vi "receiveTelemetry.vi"(8 "error in (no error)":errorcluster, 10 "tel connection in":refnum<k5>, 11 "TcpServer out":refnum<class "TcpServer.lvclass">) -> (0 "error out":errorcluster, 1 "telemetry received":string[](array[string]), 2 "tel connection out":refnum<k5>, 3 "tcpServer out":refnum<class "TcpServer.lvclass">)   [LabVIEW 2018]
doc: "Generate 50 elements and send them as telemetry to TCP client, and then read it."
uses:
  src/TcpServer/TcpServer.lvclass
  src/TcpServerTel/typedef/telTypeDef.ctl
  src/TcpServerTel/TcpServerTel.lvclass
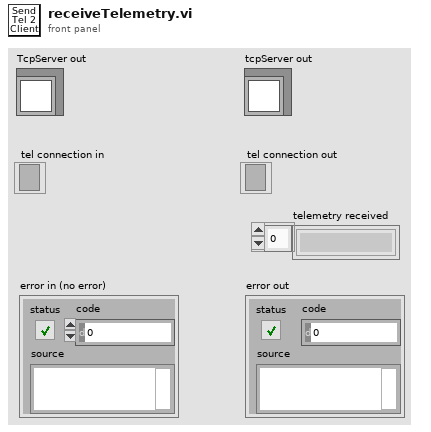
[diagram p1: front panel]
types:
  T1 = enum16{"Standard", "Buffered", "CRLF", "Immediate"}
  T2 = typedef "TcpServerTel.lvclass/telTypeDef.ctl" = cluster{"name":string, "telDetails":string}
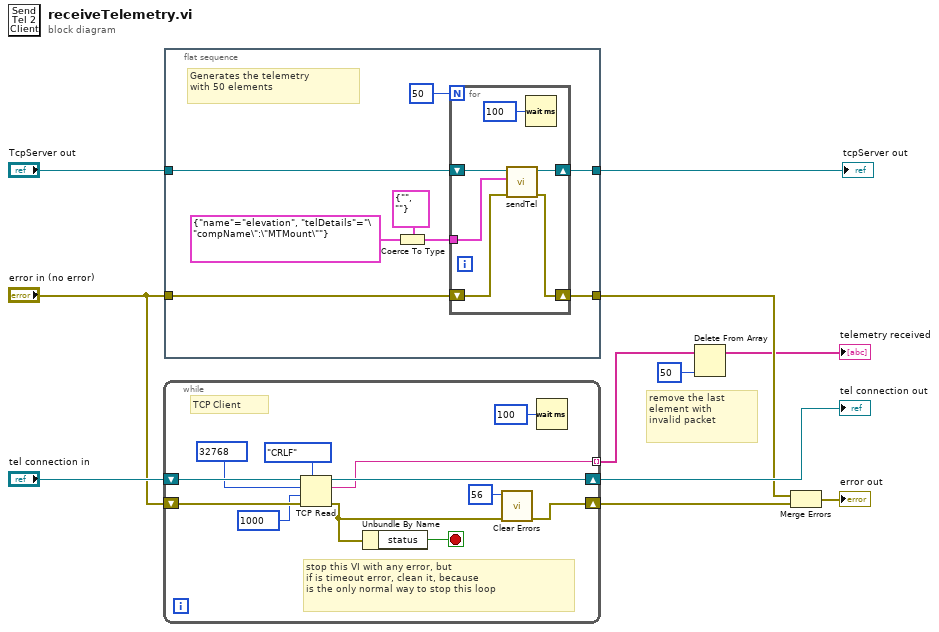
[diagram p0: block diagram]
diagram:
  # "remove the last\nelement with \ninvalid packet"
  n1 = while {
    tunnel: [w13] -> w2 mode=indexing
    shift-right: [w15] -> w6
    shift-left: "error in (no error)" -> [w21]
    shift-right: [w20] -> w11
    shift-left: "tel connection in" -> [w22]
    stop <- w12 stop-if-true
    # "stop this VI with any error, but\nif is timeout error, clean it, because\nis the only normal way to stop this loop"
    # "TCP Client"
    n2 = TCP Read(connection ID=w22, bytes to read=32768, error in (no error)=w21, 7:T1."CRLF" ("mode (standard)"), 9:1000 ("timeout ms (25000)")) -> (connection ID out=w20:refnum<k5>, data out=w13:string, error out=w16:errorcluster)
    n3 = Unbundle By Name(w16) -> ("status"=w12:bool)
    n4 = call <vilib>:"Clear Errors.vi"("error in (no error)"=w16, "specific error code to clear (0: all)"=56 ("error code (0)")) -> ("error out"=w15:errorcluster)  [unwired: 4 in, 1 out]
    n5 = Wait (ms)(milliseconds to wait=u32 100) -> ()  [unwired: 1 out]
  }
  "tel connection out" <- w11
  n6 = flat-sequence {
    tunnel: "TcpServer out" -> [w31]
    tunnel: "error in (no error)" -> [w30]
    tunnel: [w29] -> w5
    tunnel: [w24] -> w8
    frame #0 {
      # "Generates the telemetry\nwith 50 elements"
      n7 = Coerce To Type(0:T2 {"name"="elevation", "telDetails"="\"compName\":\"MTMount\""} ("x"), 1:T2 {"name"="", "telDetails"=""} ("Telemetry")) -> (2:w26:T2)
      n8 = for {
        N: 50 -> [_]
        tunnel: w26 -> [w32]
        shift-right: [w34] -> w24
        shift-left: w31 -> [w36]
        shift-right: [w37] -> w29
        shift-left: w30 -> [w35]
        n9 = call "sendTel.vi"("error in (no error)"=w35, "Telemetry"=w32, "tcpServer in"=w36) -> ("error out"=w37:errorcluster, "tcpServer out"=w34:refnum<class "TcpServer.lvclass">)  [unwired: 7 in]
        n10 = Wait (ms)(milliseconds to wait=u32 100) -> ()  [unwired: 1 out]
      }
    }
  }
  n11 = Delete From Array(array=w2, index=50) -> (array with subset deleted=→"telemetry received":string[])  [unwired: 1 in, 1 out]
  n12 = Merge Errors(w5, w6) -> (→"error out":errorcluster)
  "tcpServer out" <- w8
